vi "位置变化值监测.vi"() -> ()   [LabVIEW 2016, in "main.lvlib"]
uses:
  main.lvlib
  elevator/elevator.lvlib
panel:
  out "数组":i32[](array[numeric])
  out "位置变化值":dbl
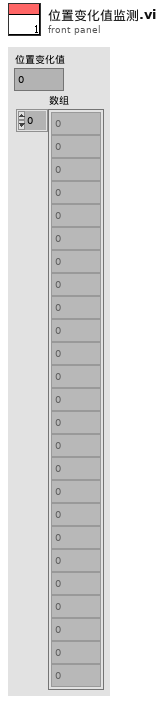
[diagram p1: front panel]
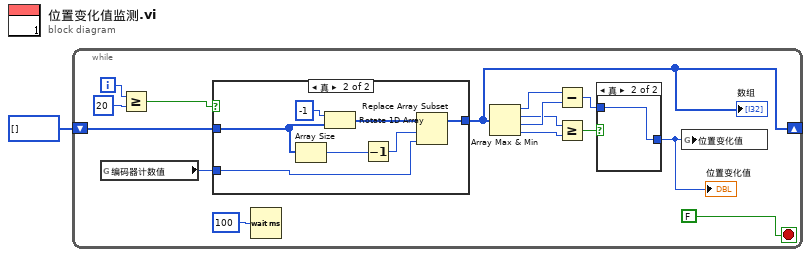
[diagram p0: block diagram]
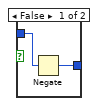
[diagram p2: hidden frame]
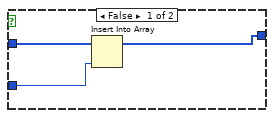
[diagram p3: hidden frame]
diagram:
  n1 = while {
    shift-right: [w11] -> _
    shift-left: i32[] [] -> [w13]
    i -> [w8]
    stop <- FALSE stop-if-true
    n2 = global read "elevator 全局变量.vi" "编码器计数值"() -> (w7:i32)
    n3 = Greater Or Equal?(x=w8, y=20) -> (x >= y?=w12:bool)
    n4 = case shown="真" w12 {
      tunnel: [w20 w29] -> w11
      tunnel: w13 -> [w22 w25]
      tunnel: w7 -> [w21 w27]
      frame False {
        n5 = Insert Into Array(array=w22, new element=w21) -> (w20:i32[])  [unwired: 1 in]
      }
      frame True {
        n6 = Array Size(array=w25) -> (size(s)=w24:i32)
        n7 = Rotate 1D Array(1:w25, 2:-1 ("n")) -> (0:w28:i32[])
        n8 = Decrement(x=w24) -> (x-1=w23:i32)
        n9 = Replace Array Subset(array=w28, new element=w27, index=w23) -> (w29:i32[])
      }
    }
    "数组" <- w11
    n10 = Wait (ms)(milliseconds to wait=u32 100 ("等待时间（毫秒）")) -> ()  [unwired: 1 out]
    n11 = Array Max & Min(array=w11) -> (max value=w10:i32, max index (indices)=w6:i32, min value=w9:i32, min index (indices)=w5:i32)
    n12 = Subtract(x=w10, y=w9) -> (x-y=w4:i32)
    n13 = Greater Or Equal?(x=w6, y=w5) -> (x >= y?=w2:bool)
    n14 = case shown="真" w2 {
      tunnel: w4 -> [w18 w19]
      tunnel: [w17 w19] -> w3
      frame False {
        n15 = Negate(x=w18) -> (-x=w17:i32)
      }
      frame True {
      }
    }
    "位置变化值" <- w3
    n16 = global write "全局非断电保持变量.vi" "位置变化值"(w3) -> ()
  }
